vi "Вывод и запись температуры.vi"() -> ()   [LabVIEW 2017]
doc: "This VI is used as a subVI in the Temperature System exercise in the LabVIEW Basics I course."
uses:
  <vilib>/Utility/file.llb/Write To Spreadsheet File (DBL).vi
panel:
  in  "Return":bool
  out "Температура":dbl(graph)
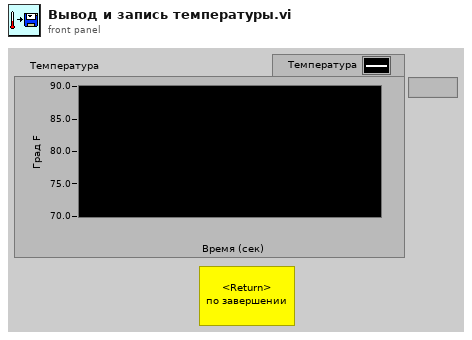
[diagram p1: front panel]
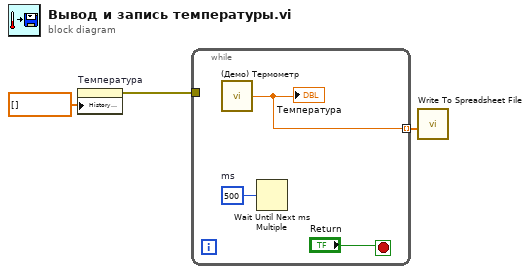
[diagram p0: block diagram]
diagram:
  n1 = property on="Температура" class="WFChart (strict)"("History Data"=dbl[] []) -> (error out=w1:errorcluster)  [unwired: 2 in, 1 out]
  n2 = while {
    tunnel: [w5] -> w3 mode=indexing
    tunnel: w1 -> [_]
    stop <- "Return" stop-if-true
    w6 = u32 500  # ms
    n3 = call "(Демо) Термометр.vi"() -> ("Температура"=w5:dbl)  [unwired: 1 in]
    "Температура" <- w5
    n4 = Wait Until Next ms Multiple(millisecond multiple=w6) -> ()  [unwired: 1 out]
  }
  n5 = call-poly <vilib>:"Write To Spreadsheet File.vi"("1D data"=w3) -> ()  [unwired: 7 in, 1 out]
